vi "Verify Arduino Libraries.vi"(8 "Error In":errorcluster, 10 "Arduino Base Path":path=path "C:/Program Files (x86)/Arduino") -> (0 "Error Out":errorcluster, 2 "Libraries Exst?":bool, 3 "Path to Arduino\\libraries":path)   [LabVIEW 2020, in "LMH-LINX.lvlib"]
uses:
  LMH-LINX.lvlib
  <vilib>/regexp/Match Regular Expression.xnode
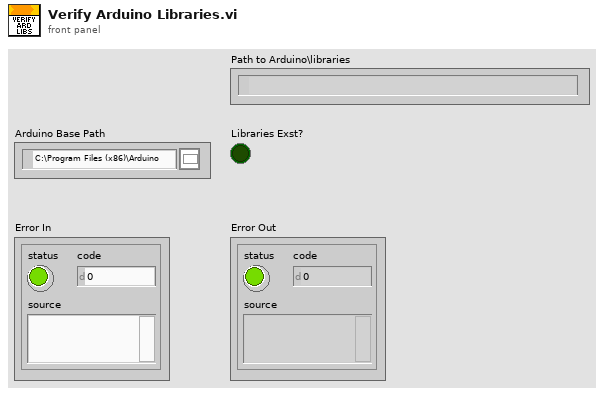
[diagram p1: front panel]
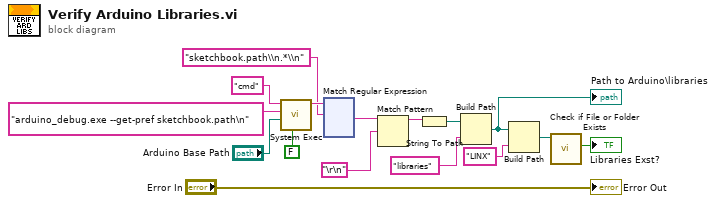
[diagram p0: block diagram]
diagram:
  n1 = call <vilib>:"System Exec.vi"("run minimized? (F)"=FALSE, "working directory"="Arduino Base Path", "standard input"="arduino_debug.exe --get-pref sketchbook.path\n", "command line"="cmd") -> ("standard output"=w12:string)  [unwired: 4 in, 3 out]
  n2 = xnode "Match Regular Expression"("input string"=w12, "regular expression"="sketchbook.path\\n.*\\n") -> ("after match"=w3:string)  [unwired: 4 in, 4 out]
  n3 = Match Pattern(string=w3, regular expression="\r\n") -> (before substring=w1:string)  [unwired: 1 in, 3 out]
  n4 = String To Path(string=w1) -> (path=w10:path)
  n5 = Build Path(base path=w10, name or relative path="libraries") -> (appended path=w8:path)
  "Path to Arduino\\libraries" <- w8
  n6 = Build Path(base path=w8, name or relative path="LINX") -> (appended path=w6:path)
  n7 = call <vilib>:"Check if File or Folder Exists.vi"("path"=w6) -> ("file or folder exists?"=→"Libraries Exst?":bool)  [unwired: 8 in, 2 out]
  "Error Out" <- "Error In"
